vi "NTV_Heartbeat.vi"(7 "Read(f) Write(t)":bool, 11 "Heartbeat":dbl) -> (3 "Heartbeat":dbl)   [LabVIEW 2020]
uses:
  <vilib>/Rock Robotics/Network Tables/NT Read Number.vi
  <vilib>/Rock Robotics/Network Tables/NT Write Number.vi
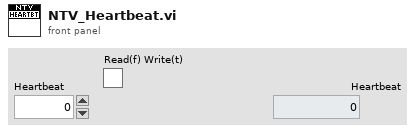
[diagram p1: front panel]
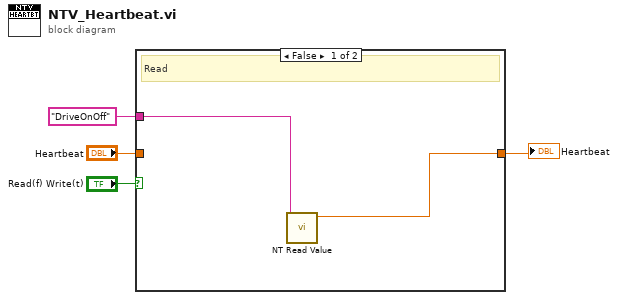
[diagram p0: block diagram]
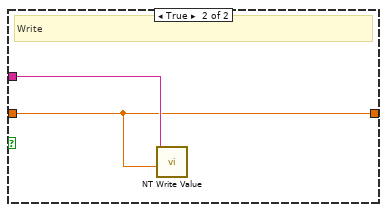
[diagram p2: hidden frame]
diagram:
  n1 = case shown="False" "Read(f) Write(t)" {
    tunnel: "Heartbeat" -> [_ w7]
    tunnel: "DriveOnOff" ("Name") -> [w6 w8]
    tunnel: [w5 w7] -> w1
    frame False {
      # "Read"
      n2 = call-poly <vilib>:"NT Read Value.vi"("name"=w6) -> ("value"=w5:dbl)  [unwired: 8 in, 2 out]
    }
    frame True {
      # "Write"
      n3 = call-poly <vilib>:"NT Write Value.vi"("value"=w7, "name"=w8) -> ()  [unwired: 9 in, 1 out]
    }
  }
  "Heartbeat" <- w1
